vi "SetPropertyAbstract.vi"(8 "error in (no error)":errorcluster, 10 "Numeric":dbl, 11 "reference in":refnum<class "G#MethodTemplates.lvclass">) -> (0 "error out":errorcluster, 3 "reference out":refnum<class "G#MethodTemplates.lvclass">)   [LabVIEW 2020, in "G#MethodTemplates.lvclass"]
uses:
  G#MethodTemplates.lvclass
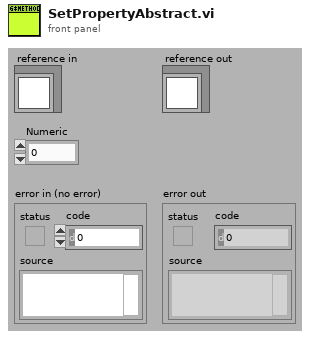
[diagram p1: front panel]
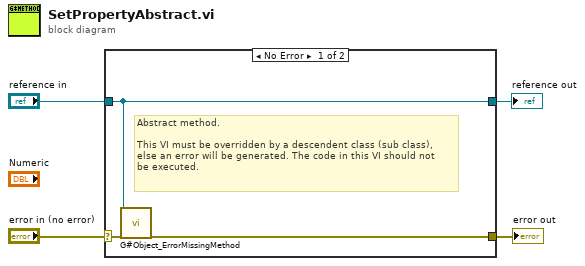
[diagram p0: block diagram]
diagram:
  n1 = case shown="No Error" "error in (no error)" {
    selector: "error in (no error)" -> [w7 w9]
    tunnel: [w6 w9] -> w4
    tunnel: [w5 w8] -> w2
    tunnel: "reference in" -> [w5 w8]
    frame No Error {
      # "Abstract method.\n\nThis VI must be overridden by a descendent class (sub class),\nelse an error will be generated. The code in this VI should not\nbe executed."
      n2 = call-dynamic "G#Object_ErrorMissingMethod.vi"("reference in"=w5, "error in (no error)"=w7) -> ("error out"=w6:errorcluster)  [unwired: 16 in, 1 out]
    }
    frame Error {
    }
  }
  "error out" <- w4
  "reference out" <- w2
